vi "uSubscription Construct.vi"(8 "error in (no error)":errorcluster, 10 "Topics":string[](array[string]), 11 "uClient_Subscriber":refnum<class "uClient_Subscriber.lvclass">) -> (0 "error out":errorcluster, 2 "Filtered Topics":string[](array[string]), 3 "uSubscriptions out":refnum<class "uSubscription.lvclass">[](array[class]))   [LabVIEW 2023, in "uLib.lvlib" / "uSubscription.lvclass"]
doc: "Pass in a list of topics and get subscriptions for the topics that conform to the subscription policy."
uses:
  uSubscription.lvclass
  uClient/uClient_Subscriber/uClient_Subscriber.lvclass
  U:/Projects/uLib/Src/uFramework/uClient/uClient.lvclass
  uClient/uClient/uClient.lvclass/uClient.ctl
  uClient/uClient_Subscriber/uClient_Subscriber.lvclass/uClient_Subscriber.ctl
  uPolicy/uPolicy/uPolicy.lvclass/uPolicy.ctl
  TypeDef_uSubscriptionPrivateData.ctl
  uNotifyMode/uNotifyMode/uNotifyMode.lvclass
  uTransport/uTransport/uTransport.lvclass
  uSubscription.lvclass/uSubscription.ctl
  uPolicy/uPolicy/Read uNotifyMode.vi
  uPolicy/uPolicy/Read uStringManipulation.vi
  uPolicy/uPolicy/uPolicy.lvclass
  uStringManipulation/uStringManipulation/uStringManipulation.lvclass
  uClient/uClient/uClient.lvclass
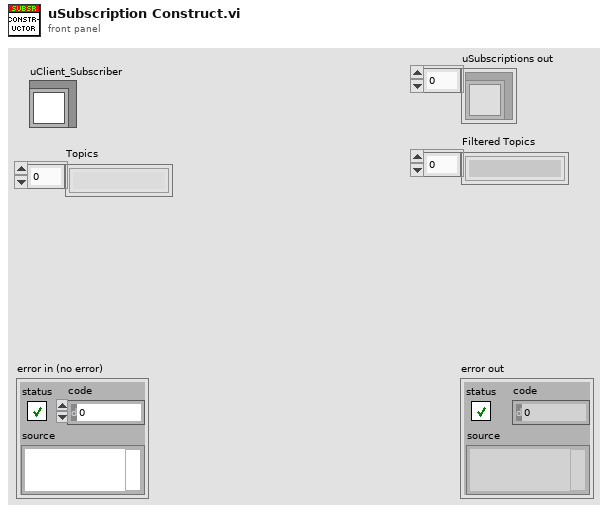
[diagram p1: front panel]
types:
  T1 = typedef "uLib.lvlib/uSubscription.lvclass/TypeDef_uSubscriptionPrivateData.ctl" = cluster{"Destination CMD":string, "uNotifyMode":refnum<class "uNotifyMode.lvclass">, "Destination uTransport":refnum<class "uTransport.lvclass">}
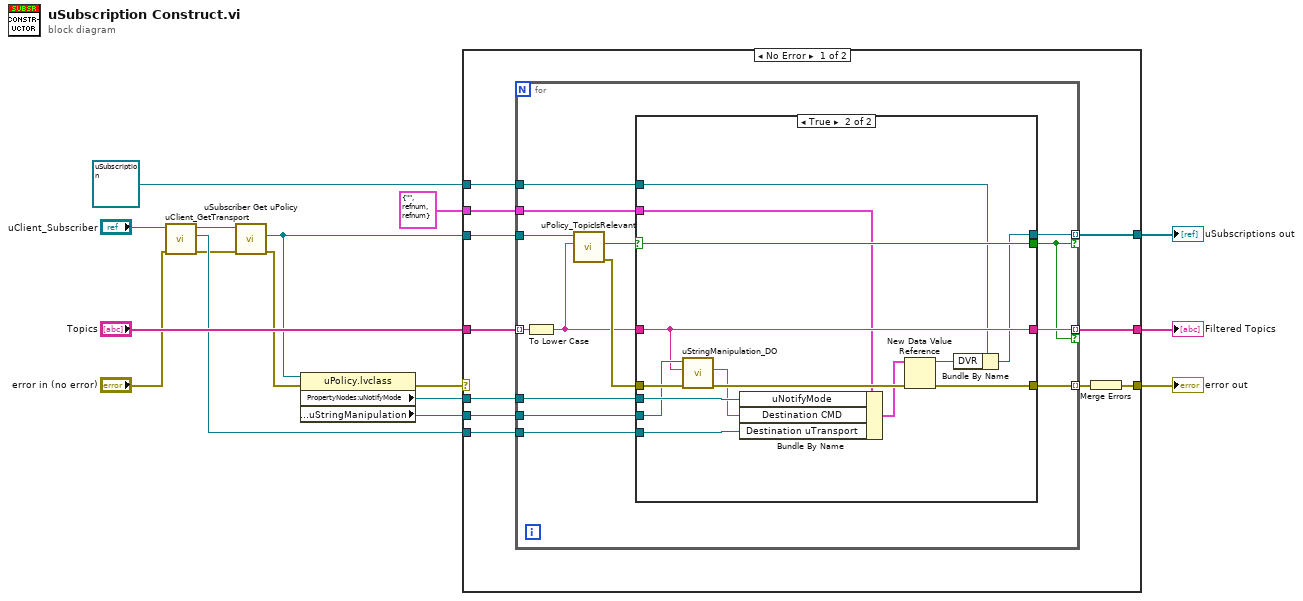
[diagram p0: block diagram]
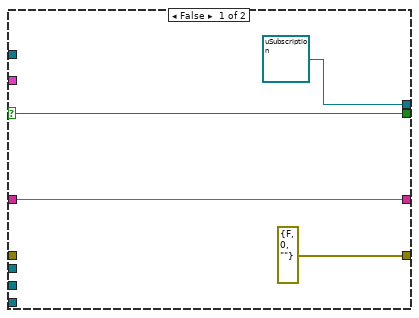
[diagram p2: hidden frame]
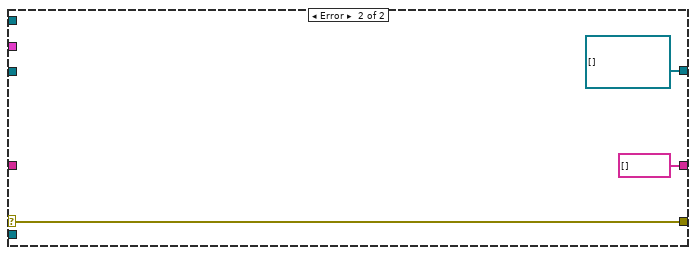
[diagram p3: hidden frame]
diagram:
  n1 = call "uClient_GetTransport.vi"("error in (no error)"="error in (no error)", "uClient in"="uClient_Subscriber") -> ("error out"=w5:errorcluster, "uTransport"=w7:refnum<class "uTransport.lvclass">, "uClient out"=w6:refnum<class "uClient_Subscriber.lvclass">)  [unwired: 7 in]
  n2 = call "uSubscriber Get uPolicy.vi"("error in (no error)"=w5, "uClient_Subscriber in"=w6) -> ("error out"=w4:errorcluster, "uPolicy"=w3:refnum<class "uPolicy.lvclass">)  [unwired: 7 in, 1 out]
  n3 = property class="uPolicy.lvclass"(reference=w3, error in=w4) -> (error out=w11:errorcluster, "PropertyNodes:uNotifyMode"=w12:refnum<class "uNotifyMode.lvclass">, "PropertyNodes:uStringManipulation"=w13:refnum<class "uStringManipulation.lvclass">)  [unwired: 1 out]
  n4 = case shown="No Error" w11 {
    selector: w11 -> [_ w62]
    tunnel: refnum<class "uSubscription.lvclass"> refnum ("uSubscription in") -> [w27 _]
    tunnel: "Topics" -> [w26 _]
    tunnel: [w21 w62] -> w14
    tunnel: w13 -> [w25 _]
    tunnel: w12 -> [w24 _]
    tunnel: w3 -> [w23 _]
    tunnel: [w20 refnum<class "uSubscription.lvclass">[] []] -> w10
    tunnel: w7 -> [w19 _]
    tunnel: [w18 string[] []] -> w2
    tunnel: T1 {"Destination CMD"="", "uNotifyMode"=refnum, "Destination uTransport"=refnum} ("uSubscription") -> [w17 _]
    frame No Error {
      n5 = for {
        tunnel: w27 -> [w40]
        tunnel: w26 -> [w37] mode=indexing
        tunnel: w25 -> [w36]
        tunnel: w24 -> [w39]
        tunnel: w23 -> [w38]
        tunnel: [w35] -> w22 mode=indexing
        tunnel: [w33] -> w20 mode=indexing if=w30
        tunnel: w19 -> [w32]
        tunnel: [w31] -> w18 mode=indexing if=w30
        tunnel: w17 -> [w28]
        n6 = To Lower Case(string=w37) -> (all lower case string=w29:string)
        n7 = call-dynamic "uPolicy_TopicIsRelevant.vi"("Observed Topic (Lower Case)"=w29, "uPolicy_All in"=w38) -> ("error out"=w41:errorcluster, "Relevant?"=w34:bool)  [unwired: 7 in, 1 out]
        n8 = case shown="True" w34 {
          selector: w34 -> [w43 w54]
          tunnel: w40 -> [_ w49]
          tunnel: w39 -> [_ w57]
          tunnel: w29 -> [w42 w52]
          tunnel: w36 -> [_ w55]
          tunnel: [errorcluster {"status"=FALSE, "code"=0, "source"=""} ("error out") w51] -> w35
          tunnel: w41 -> [_ w59]
          tunnel: [refnum<class "uSubscription.lvclass"> refnum ("uSubscription in") w47] -> w33
          tunnel: [w43 w54] -> w30
          tunnel: w32 -> [_ w53]
          tunnel: [w42 w52] -> w31
          tunnel: w28 -> [_ w46]
          frame False {
          }
          frame True {
            n9 = call-dynamic "uStringManipulation_DO.vi"("error in (no error)"=w59, "String in"=w52, "uStringManipulation in"=w55) -> ("error out"=w58:errorcluster, "String"=w56:string)  [unwired: 6 in, 1 out]
            n10 = Bundle By Name(cluster=w46, "uNotifyMode"=w57, "Destination CMD"=w56, "Destination uTransport"=w53) -> (w50:T1)
            n11 = New Data Value Reference(data value=w50, error in=w58) -> (data value reference=w48:refnum<data-value>, error out=w51:errorcluster)
            n12 = Bundle By Name(cluster=w49, "DVR"=w48) -> (w47:refnum<class "uSubscription.lvclass">)
          }
        }
      }
      n13 = Merge Errors(w22) -> (w21:errorcluster)
    }
    frame Error {
    }
  }
  "error out" <- w14
  "uSubscriptions out" <- w10
  "Filtered Topics" <- w2
